vi "第四题.vi"() -> ()   [LabVIEW 2017]
uses:
  <vilib>/Analysis/2dsp.llb/Real FFT.vi
  <vilib>/Analysis/NI_AALPro.lvlib
  <vilib>/measure/NI_MABase.lvlib
panel:
  in  "amplitude 3":dbl=1.0 format="%0.2p"
  in  "frequency 3":dbl=10.0 caption="频率3" format="%0.2p"
  in  "amplitude 2":dbl=1.0 caption="幅值2" format="%0.2p"
  in  "frequency 2":dbl=10.0 caption="频率2" format="%0.2p"
  in  "amplitude":dbl=1.0 caption="幅值1" format="%0.2p"
  in  "frequency":dbl=10.0 caption="频率1" format="%0.2p"
  out "时域信号":dbl[](graph)
  out "频域信号":dbl[](graph)
  # "幅值3"
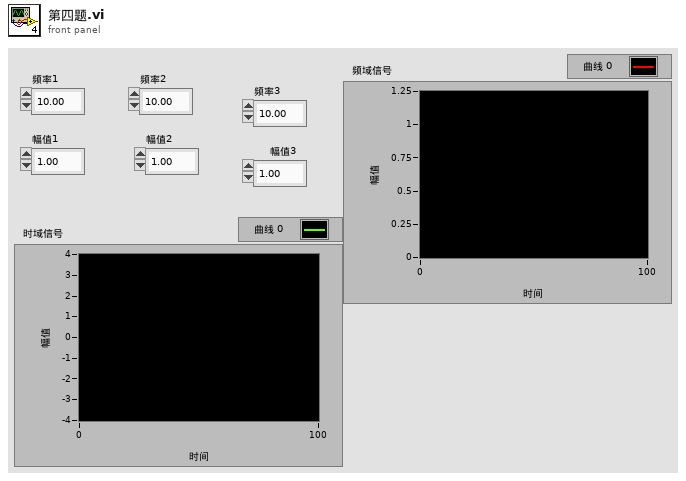
[diagram p1: front panel]
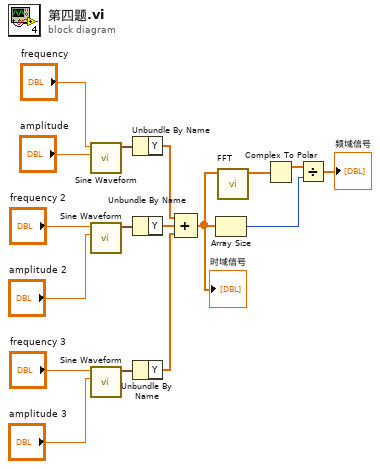
[diagram p0: block diagram]
diagram:
  n1 = call <vilib>:"Sine Waveform.vi"("amplitude"="amplitude", "frequency"="frequency") -> ("signal out"=w13:waveform(dbl))  [unwired: 8 in, 1 out]
  n2 = call <vilib>:"Sine Waveform.vi"("amplitude"="amplitude 2", "frequency"="frequency 2") -> ("signal out"=w12:waveform(dbl))  [unwired: 8 in, 1 out]
  n3 = call <vilib>:"Sine Waveform.vi"("amplitude"="amplitude 3", "frequency"="frequency 3") -> ("signal out"=w11:waveform(dbl))  [unwired: 8 in, 1 out]
  n4 = Unbundle By Name(w13) -> ("Y"=w9:dbl[])
  n5 = Unbundle By Name(w12) -> ("Y"=w10:dbl[])
  n6 = Unbundle By Name(w11) -> ("Y"=w8:dbl[])
  n7 = Compound Arithmetic op=ADD(w9, w10, w8) -> (w7:dbl[])
  "时域信号" <- w7
  n8 = Array Size(array=w7) -> (size(s)=w15:i32)
  n9 = call-poly <vilib>:"FFT.vi"("X"=w7) -> ("FFT {X}"=w14:cdb[])  [unwired: 9 in, 1 out]
  n10 = Complex To Polar(r * e^(i*theta)=w14) -> (r=w16:dbl[])  [unwired: 1 out]
  n11 = Divide(x=w16, y=w15) -> (x/y=→"频域信号":dbl[])
